vi "Read Trigger Interface.vi"(8 "error in (no error)":errorcluster, 11 "Control_interface in":refnum<class "Control_interface.lvclass">) -> (0 "error out":errorcluster, 2 "Trigger Interface":T1={"Slope"=0, "Level"=30, "Source"=0, "External Range"=2000, "External Coupling"=0, "External"=TRUE, "Disable"=FALSE, "External Impedance"=1} {"External Impedance" items=["50 Ohm", "HiZ"]; "External Coupling" items=["DC", "AC"]; "External Range" min=2000 max=10000 step=8000; "Slope" items=["Rising", "Falling"]; "Level" min=-100 max=100; "Source" min=0 max=64 step=1}, 3 "Control_interface out":refnum<class "Control_interface.lvclass">)   [LabVIEW 2015, in "Control_interface.lvclass"]
uses:
  Control_interface.lvclass
  Control_interface.lvclass/Control_interface.ctl
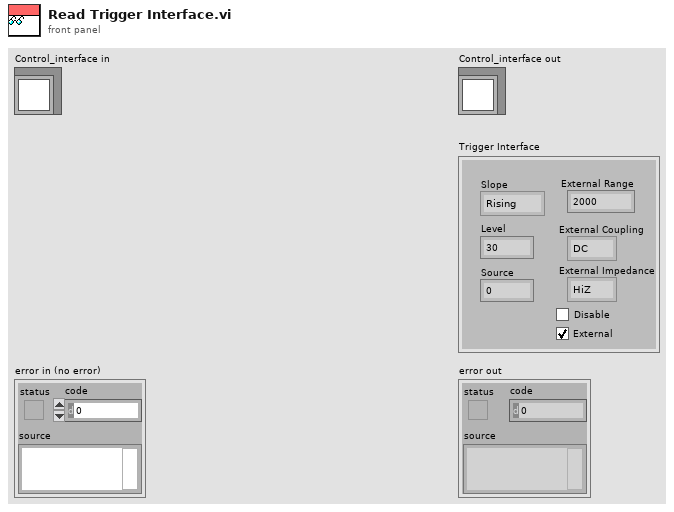
[diagram p1: front panel]
types:
  T1 = cluster{"Slope":u16, "Level":i32, "Source":i32, "External Range":u32, "External Coupling":u16, "External":bool, "Disable":bool, "External Impedance":u16}
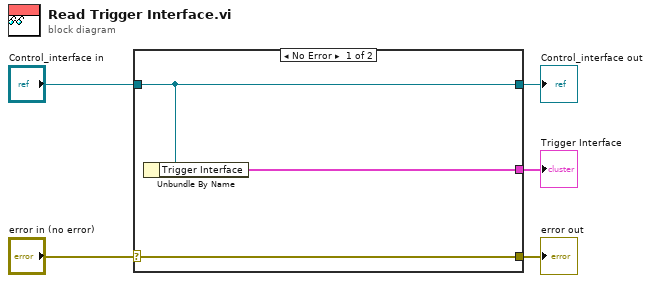
[diagram p0: block diagram]
diagram:
  n1 = case shown="No Error" "error in (no error)" {
    selector: "error in (no error)" -> [w8 w9]
    tunnel: [w8 w9] -> w4
    tunnel: [w7 w10] -> w2
    tunnel: "Control_interface in" -> [w7 w10]
    tunnel: [w6 _] -> w1
    frame No Error {
      n2 = Unbundle By Name(w7) -> ("Trigger Interface"=w6:T1)
    }
    frame Error {
    }
  }
  "error out" <- w4
  "Control_interface out" <- w2
  "Trigger Interface" <- w1
